vi "oa_STFT Spectrogram at Indices (Even-angle).vi"(0 "even-angle signal":cluster{"r0":dbl, "dr":dbl, "Y":dbl[]}={"r0"=0.0, "dr"=1.0, "Y"=[]} {"r0" format="%.2p"; "dr" format="%.2p"; "Y" format="%.2f"}, 3 "reset? (True)":bool=TRUE, 5 "rev indices":dbl[](array[numeric]) format="%.2f", 7 "X scale in":cluster{"offset":dbl, "multiplier":dbl} {"multiplier" format="%.2f"; "offset" format="%.2f"}, 9 "last indices":dbl format="%.2f", 11 "error in (no error)":errorcluster, 12 "spectral settings":T2={"window type"=1, "number of lines"=400} {"number of lines" min=2; "window type" items=["None"=0, "Hanning"=1, "Hamming"=2, "Blackman-Harris"=3, "Exact Blackman"=4, "Blackman"=5, "Flat Top"=6, "4 Term B-Harris"=7, "7 Term B-Harris"=8, "Low Sidelobe"=9, "Gaussian"=62]}) -> (4 "spectral map":dbl[][](array[numeric]) format="%.2f", 6 "scales":T1 {"Y scale"."multiplier" format="%.2f"; "Y scale"."offset" format="%.2f"; "X scale"."multiplier" format="%.2f"; "X scale"."offset" format="%.2f"}, 14 "finished":bool, 15 "error out":errorcluster)   [LabVIEW 2017, in "SoundVib_Resampling.lvlib"]
doc: "Computes Short Time Fourier Transform spectrogram at specified indices."
uses:
  <vilib>/addons/Sound and Vibration/Order Analysis/Resample Order Tracking/SoundVib_Resampling.lvlib
  <vilib>/Analysis/NI_AALPro.lvlib
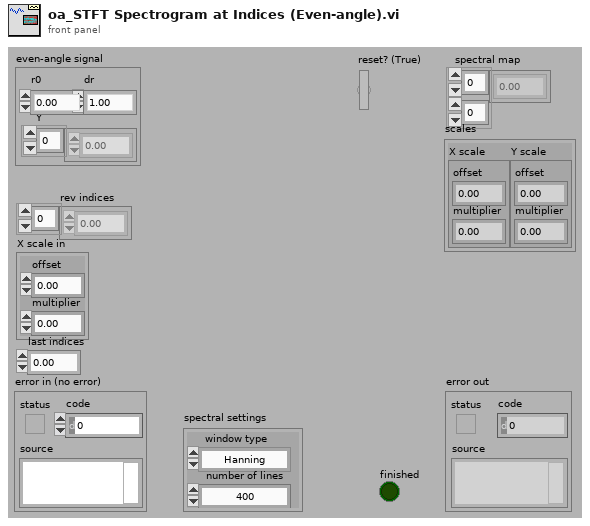
[diagram p1: front panel]
types:
  T1 = cluster{"X scale":cluster{"offset":dbl, "multiplier":dbl}, "Y scale":cluster{"offset":dbl, "multiplier":dbl}}
  T2 = cluster{"window type":u32, "number of lines":i32}
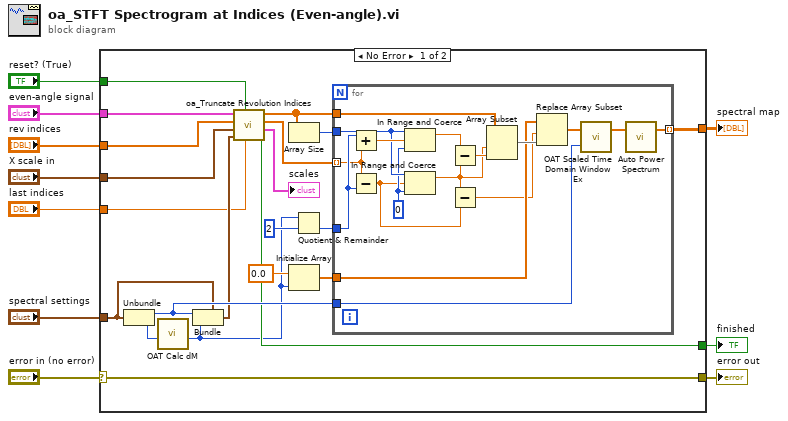
[diagram p0: block diagram]
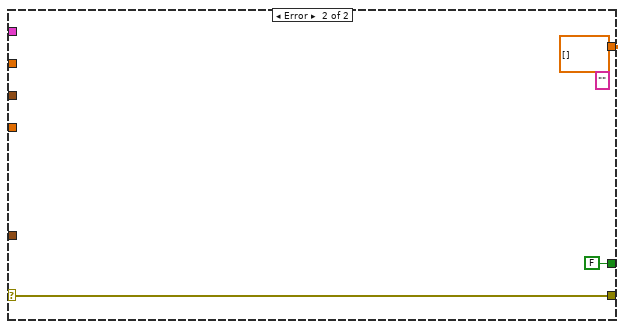
[diagram p2: hidden frame]
diagram:
  n1 = case shown="No Error" "error in (no error)" {
    selector: "error in (no error)" -> [w13 w51]
    tunnel: [w12 dbl[][] [] ("log view [dB EU]")] -> w10
    tunnel: "rev indices" -> [w26 _]
    tunnel: "even-angle signal" -> [w11 _]
    tunnel: "spectral settings" -> [w22 _]
    tunnel: "reset? (True)" -> [w21 _]
    tunnel: [w19 FALSE ("finished")] -> w5
    tunnel: "X scale in" -> [w18 _]
    tunnel: "last indices" -> [w14 _]
    tunnel: [w13 w51] -> w1
    frame No Error {
      n2 = Unbundle(w22) -> ("window type"=w23:u32, "number of lines"=w24:i32)
      n3 = call <vilib>:"OAT Calc dM.vi"("window length"=w24) -> ("actual window length"=w16:i32)  [unwired: 7 in, 3 out]
      n4 = Bundle(cluster=w22, "window type"=w23, "number of lines"=w16) -> (w17:T2)
      n5 = call <vilib>:"oa_Truncate Revolution Indices.vi"("last indices"=w14, "reset? (True)"=w21, "spectral settings"=w17, "X scale in"=w18, "rev in"=w26, "even-angle signal"=w11) -> ("finished"=w19:bool, "scales"=→"scales":T1, "window indices"=w20:dbl[], "data out"=w25:dbl[])  [unwired: 2 in]
      n6 = Array Size(array=w25) -> (size(s)=w29:i32)
      n7 = Initialize Array(0.0 ("Element Data"), w16) -> (w27:dbl[])
      n8 = Quotient & Remainder(x=w16, y=2) -> (floor(x/y)=w30:i32)  [unwired: 1 out]
      n9 = for {
        tunnel: w25 -> [w39]
        tunnel: w20 -> [w47] mode=indexing
        tunnel: w30 -> [w48]
        tunnel: w29 -> [w45]
        tunnel: w27 -> [w37]
        tunnel: w23 -> [w33]
        tunnel: [w32] -> w12 mode=indexing
        w44 = 0 ("lower limit")
        n10 = Add(x=w48, y=w47) -> (x+y=w46:dbl)
        n11 = Subtract(x=w47, y=w48) -> (x-y=w42:dbl)
        n12 = In Range and Coerce(upper limit=w45, x=w46, lower limit=w44) -> (coerced(x)=w43:dbl)  [unwired: 1 out]
        n13 = In Range and Coerce(upper limit=w45, x=w42, lower limit=w44) -> (coerced(x)=w40:dbl)  [unwired: 1 out]
        n14 = Subtract(x=w43, y=w40) -> (x-y=w41:dbl)
        n15 = Subtract(x=w40, y=w42) -> (x-y=w36:dbl)
        n16 = Array Subset(array=w39, index=w40, length=w41) -> (w38:dbl[])
        n17 = Replace Array Subset(array=w37, new element=w38, index=w36) -> (w35:dbl[])
        n18 = call <vilib>:"OAT Scaled Time Domain Window Ex.vi"("window type"=w33, "X"=w35) -> ("y"=w34:dbl[])  [unwired: 1 out]
        n19 = call <vilib>:"Auto Power Spectrum.vi"("Signal (V)"=w34) -> ("Power Spectrum (V^2 rms)"=w32:dbl[])  [unwired: 1 in, 1 out]
      }
    }
    frame Error {
      (unwired) "" ("unit label")
    }
  }
  "spectral map" <- w10
  "finished" <- w5
  "error out" <- w1
